vi "UHR-Fleezers Control (host) -Leonardo 04-2018 V2_sym.vi"(0 "Tab Control":T5(tab)=enum."Trap Control (RF)") -> ()   [LabVIEW 2013] (continued)
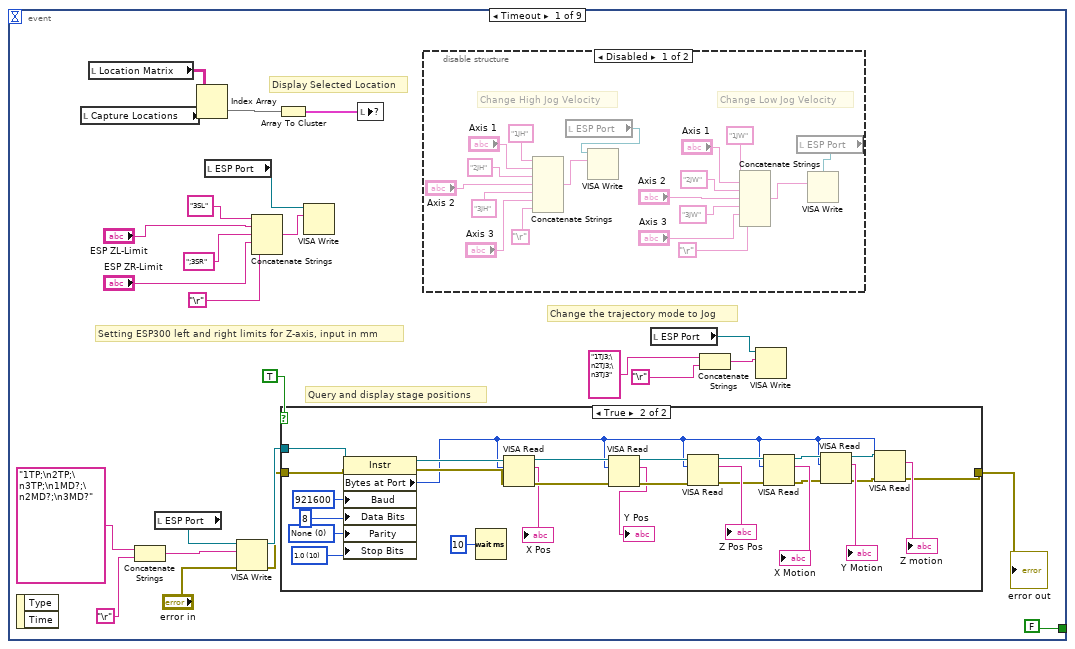
[diagram p2: hidden frame]
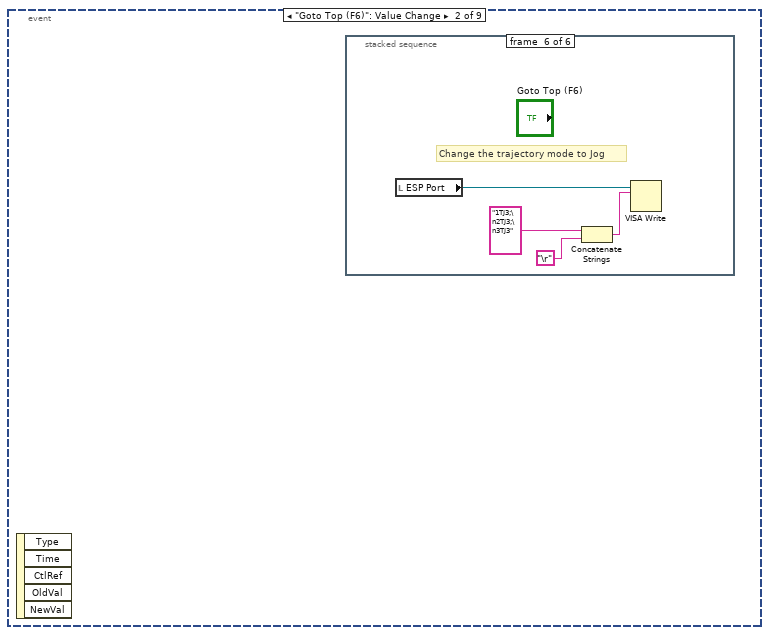
[diagram p5: hidden frame]
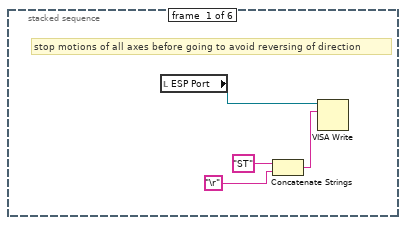
[diagram p6: hidden frame]
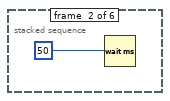
[diagram p7: hidden frame]
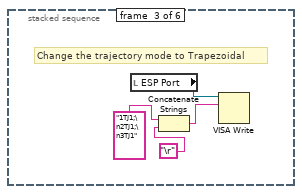
[diagram p8: hidden frame]
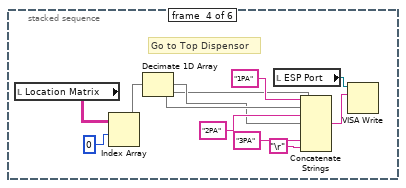
[diagram p9: hidden frame]
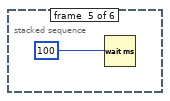
[diagram p10: hidden frame]
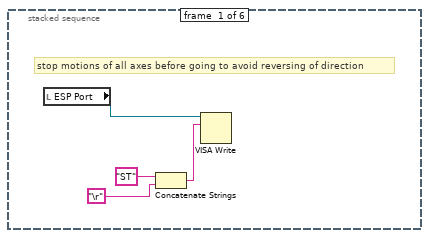
[diagram p11: hidden frame]
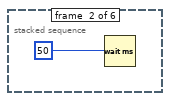
[diagram p12: hidden frame]
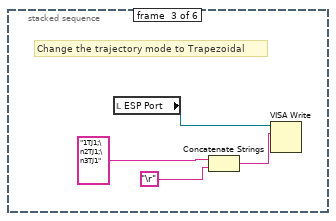
[diagram p13: hidden frame]
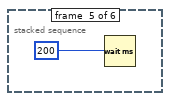
[diagram p14: hidden frame]
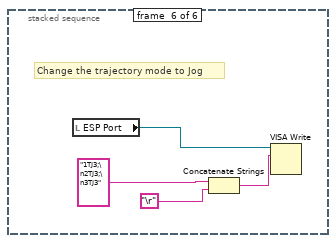
[diagram p15: hidden frame]
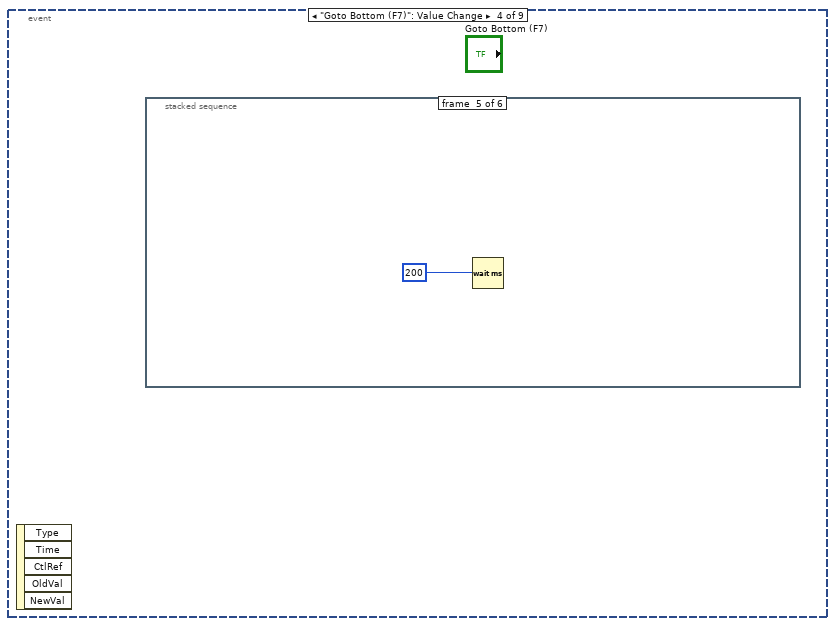
[diagram p16: hidden frame]
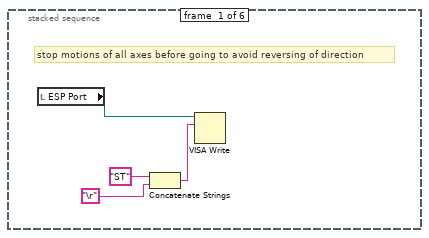
[diagram p17: hidden frame]
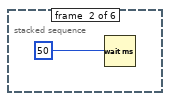
[diagram p18: hidden frame]
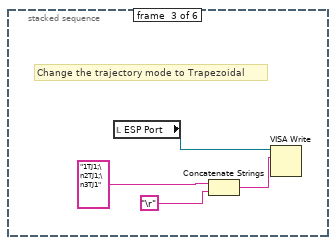
[diagram p19: hidden frame]
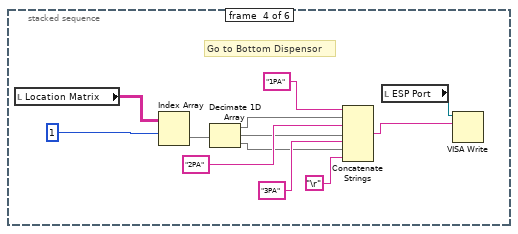
[diagram p20: hidden frame]
                    n2323 = Write to Binary File(file (use dialog)=w3981, data=w3980, 5:FALSE ("prepend array or string size? (T)"), 9:T30."big-endian, network order" ("byte order (0:big-endian, network order)")) -> ()  [unwired: 1 in, 4 out]
                  }
                }
                n2324 = Greater?(x="Save ave N", y=1.0) -> (0:w3950:bool)
                n2325 = Not(x=w3947) -> (.not. x?=w3949:bool)
                n2326 = And(x=w3949, y=w3950) -> (x .and. y?=w3892:bool)
                n2327 = case shown="True" w3892 {
                  tunnel: w3891 -> [w3961 w3972]
                  tunnel: [w3961 w3964] -> w3890
                  tunnel: "Save ave N" -> [_ w3965]
                  frame False {
                  }
                  frame True {
                    w3962 = 2 ("dimension size")
                    n2328 = Array Size(array=w3972) -> (size(s)=w3966:i32)
                    n2329 = Divide(x=w3966, y=w3962) -> (x/y=w3970:dbl)
                    n2330 = Reshape Array(w3972, w3970, w3962) -> (w3971:u64[][])
                    n2331 = Transpose 2D Array(2D array=w3971) -> (transposed array=w3969:u64[][])
                    n2332 = for {
                      tunnel: w3969 -> [w3974] mode=indexing
                      tunnel: [w3973] -> w3963 mode=indexing
                      tunnel: w3965 -> [w3975]
                      workers-P: _ -> [_]
                      n2333 = call "downsample 1D array - U64.vi"("Ave N"=w3975, "Array In"=w3974) -> ("Array Out"=w3973:u64[])  [unwired: 1 in]
                    }
                    n2334 = Transpose 2D Array(2D array=w3963) -> (transposed array=w3968:u64[][])
                    n2335 = Divide(x=w3966, y=w3965) -> (x/y=w3967:dbl)
                    n2336 = Reshape Array(w3968, w3967) -> (w3964:u64[])
                  }
                }
                n2337 = case shown="True" w3892 {
                  tunnel: w3952 -> [w3984 w3996]
                  tunnel: [w3984 w3988] -> w3948
                  tunnel: "Save ave N" -> [_ w3989]
                  tunnel: w3943 -> [_ w3987]
                  frame False {
                    # "don't downsample data for trap calibration"
                  }
                  frame True {
                    n2338 = Array Size(array=w3996) -> (size(s)=w3990:i32)
                    n2339 = Array Size(array=w3987) -> (size(s)=w3986:i32)
                    n2340 = Divide(x=w3990, y=w3986) -> (x/y=w3994:dbl)
                    n2341 = Reshape Array(w3996, w3994, w3986) -> (w3995:i16[][])
                    n2342 = Transpose 2D Array(2D array=w3995) -> (transposed array=w3993:i16[][])
                    n2343 = for {
                      tunnel: w3993 -> [w3999] mode=indexing
                      tunnel: [w3998] -> w3985 mode=indexing
                      tunnel: w3989 -> [w3997]
                      workers-P: _ -> [_]
                      n2344 = call "downsample 1D array - I16.vi"("Ave N"=w3997, "Array In"=w3999) -> ("Array Out"=w3998:i16[])  [unwired: 1 out]
                    }
                    n2345 = Transpose 2D Array(2D array=w3985) -> (transposed array=w3992:i16[][])
                    n2346 = Divide(x=w3990, y=w3989) -> (x/y=w3991:dbl)
                    n2347 = Reshape Array(w3992, w3991) -> (w3988:i16[])
                  }
                }
                n2348 = Index Array(array=w3914, index=1) -> (element=w3917:waveform(dbl))
                n2349 = Index Array(array=w3914, index=0) -> (element=w3919:waveform(dbl))
                n2350 = Unbundle By Name(w3917) -> ("Y"=w3921:dbl[])
                n2351 = Unbundle By Name(w3919) -> ("Y"=w3929:dbl[])
                n2352 = case "Write trap pos. data" shown="True" w3895 {
                  tunnel: w3894 -> [_ w3977]
                  tunnel: w3890 -> [_ w3976]
                  frame False {
                  }
                  frame True {
                    n2353 = Write to Binary File(file (use dialog)=w3977, data=w3976, 5:FALSE ("prepend array or string size? (T)"), 9:T30."big-endian, network order" ("byte order (0:big-endian, network order)")) -> ()  [unwired: 1 in, 4 out]
                  }
                }
                n2354 = Write to Binary File(file (use dialog)=w3955, data=w3948, 5:FALSE ("prepend array or string size? (T)"), 9:T30."big-endian, network order" ("byte order (0:big-endian, network order)")) -> ()  [unwired: 1 in, 4 out]
                n2355 = feedback #26(w3921) -> (w3923:dbl[])
                n2356 = Build Array (concatenate)(w3923, w3921) -> (w3922:dbl[])
                n2357 = Select(t=w3921, s=w3897, f=w3922) -> (s? t:f=w3907:dbl[])
                n2358 = feedback-in #26(w3907) -> ()
                n2359 = feedback #27(w3929) -> (w3942:dbl[])
                n2360 = Build Array (concatenate)(w3942, w3929) -> (w3941:dbl[])
                n2361 = Select(t=w3929, s=w3897, f=w3941) -> (s? t:f=w3916:dbl[])
                n2362 = feedback-in #27(w3916) -> ()
                n2363 = Divide(x=w3956, y=w3957) -> (x/y=w3959:dbl)
                n2364 = Multiply(x=w3959, y=100.0) -> (x*y=w3958:dbl)
                n2365 = Build Array(w3916, w3907) -> (→"Saved APD":dbl[][])
                n2366 = Array Size(array=w3916) -> (size(s)=w3934:i32)
                n2367 = Unbundle By Name(w3936) -> ("Y"=w3940:dbl[])
                n2368 = Subtract(x=w3934, y="N pts to average") -> (x-y=w3910:i32)
                n2369 = Multiply(x="N pts to average", y=u16 2) -> (x*y=w3911:u16)
                n2370 = Subtract(x=w3934, y=w3911) -> (x-y=w3909:i32)
                n2371 = feedback #28(w3940) -> (w3939:dbl[])
                n2372 = Build Array (concatenate)(w3939, w3940) -> (w3938:dbl[])
                n2373 = Select(t=w3940, s=w3897, f=w3938) -> (s? t:f=w3937:dbl[])
                "Trap Delta Graph" <- w3937
                n2374 = feedback-in #28(w3937) -> ()
                n2375 = Array Subset(array=w3916, index=w3910, length="N pts to average") -> (w3933:dbl[])
                n2376 = Array Subset(array=w3916, index=w3909, length="N pts to average") -> (w3932:dbl[])
                n2377 = Array Subset(array=w3907, index=w3910, length="N pts to average") -> (w3913:dbl[])
                n2378 = Array Subset(array=w3907, index=w3909, length="N pts to average") -> (w3912:dbl[])
                n2379 = call-poly <vilib>:"Mean.vi"("X"=w3933) -> ("mean"=w3931:dbl)  [unwired: 1 out]
                n2380 = call-poly <vilib>:"Mean.vi"("X"=w3913) -> ("mean"=w3906:dbl)  [unwired: 1 out]
                n2381 = call-poly <vilib>:"Mean.vi"("X"=w3932) -> ("mean"=w3930:dbl)  [unwired: 1 out]
                n2382 = call-poly <vilib>:"Mean.vi"("X"=w3912) -> ("mean"=w3905:dbl)  [unwired: 1 out]
                n2383 = Subtract(x=w3906, y=w3905) -> (x-y=w3896:dbl)
                "Delta Fl. 2" <- w3896
                n2384 = Subtract(x=w3931, y=w3930) -> (x-y=w3928:dbl)
                "Delta Fl. 1" <- w3928
                n2385 = Initialize Array(w3928, 1 ("dimension size")) -> (w3925:dbl[])
                n2386 = Initialize Array(w3896, 1 ("dimension size")) -> (w3902:dbl[])
                n2387 = feedback #29(w3925) -> (w3926:dbl[])
                n2388 = Build Array (concatenate)(w3926, w3925) -> (w3924:dbl[])
                n2389 = feedback #30(w3902) -> (w3903:dbl[])
                n2390 = Build Array (concatenate)(w3903, w3902) -> (w3901:dbl[])
                n2391 = Select(t=w3925, s=w3897, f=w3924) -> (s? t:f=w3900:dbl[])
                n2392 = feedback-in #29(w3900) -> ()
                n2393 = Select(t=w3902, s=w3897, f=w3901) -> (s? t:f=w3899:dbl[])
                n2394 = feedback-in #30(w3899) -> ()
                n2395 = Build Array(w3900, w3899) -> (→"Save APD Deriv":dbl[][])
              }
            }
            "Progress" <- w3873
            "Progress 2" <- w3873
          }
        }
      }
    }
    n2396 = Divide(x=w2254, y=w2255) -> (x/y=w2245:ext)
    "Trap 2 amplitude" <- w2245
    n2397 = Bundle By Name(cluster=w2508, "Green FB Ch 0"=w2507, "Green FB Ch 1"=w2506) -> (w2492:T49)
    "Green FB Signals (V)" <- w2492
    n2398 = case shown="True" w2247 {
      tunnel: w2246 -> [_ w2597]
      tunnel: w2245 -> [_ w2596]
      frame False {
      }
      frame True {
        w2598 = 50.0
        n2399 = Greater?(x=w2596, y=w2598) -> (0:w2594:bool)
        n2400 = Greater?(x=w2597, y=w2598) -> (0:w2595:bool)
        n2401 = Or(x=w2595, y=w2594) -> (x .or. y?=w2593:bool)
        n2402 = case shown="True" w2593 {
          frame False {
          }
          frame True {
            n2403 = property on="All FB On/Off" class="Bool (strict)"("Val(Sgnl)"=FALSE) -> ()  [unwired: 2 in, 2 out]
            "Feedback overload" <- TRUE
          }
        }
      }
    }
    n2404 = Unbundle By Name(w2492) -> ("Green FB Ch 2"=→"Green FB Plot":dbl)
    n2405 = local read "wait to reset values"() -> (w2576:bool)
    n2406 = Not(x=w2573) -> (.not. x?=w2577:bool)
    n2407 = And(x=w2577, y=w2576) -> (x .and. y?=w2578:bool)
    n2408 = case "Part of MCL raster scanning: returns to initial positions after scan done" shown="True" w2578 {
      tunnel: w2581 -> [w3422 w3429]
      tunnel: [w3422 w3428] -> w2580
      tunnel: w2575 -> [w3421 w3427]
      tunnel: [w3421 w3426] -> w2574
      frame False {
      }
      frame True {
        w3437 = 10.0 ("y")
        w3436 = 32767.0 ("y")
        # "to return scan values\nafter a synchronous \nAOM scan"
        n2409 = local read "AO2"() -> (w3430:dbl)
        n2410 = local read "AO1"() -> (w3431:dbl)
        n2411 = local write "wait to reset values"(FALSE ("wait to reset values")) -> ()
        n2412 = Multiply(x=w3431, y=w3436) -> (x*y=w3433:dbl)
        n2413 = Multiply(x=w3430, y=w3436) -> (x*y=w3435:dbl)
        n2414 = Divide(x=w3433, y=w3437) -> (x/y=w3432:dbl)
        n2415 = Divide(x=w3435, y=w3437) -> (x/y=w3434:dbl)
        n2416 = To Word Integer(number=w3432) -> (16bit integer=w3438:i16)
        n2417 = To Word Integer(number=w3434) -> (16bit integer=w3439:i16)
        n2418 = local read "Total Counts (ticks)"() -> (w3423:u32)
        n2419 = xnode "Read/Write Control"("FPGA VI Reference In"=w3429, "error in"=w3427, "AO1 (Y)"=w3438, "AO2 (X)"=w3439, "MCL count"=w3423) -> ("FPGA VI Reference Out"=w3428:T20, "error out"=w3426:errorcluster)
        n2420 = local read "Scan Range (V)\n(of steps)"() -> (w3424:dbl)
        n2421 = property on="Scan Range (V)\n(of steps)" class="DigNum (strict)"("Val(Sgnl)"=w3424) -> ()  [unwired: 2 in, 2 out]
      }
    }
    n2422 = node-c288() -> ()  [unwired: 2 out]
  }
  n2423 = node-c288(3 ("Processor")) -> (w108:T25)  [unwired: 3 out]
  n2424 = timed-loop "Oscillate AOD (debugging)" {
    tunnel: w61 -> [w4001]
    tunnel: [w4000] -> w72
    timing: w108 -> [_]
    timing-out: [_] -> w107
    stop <- w4000 stop-if-true
    n2425 = node-c288() -> ()  [unwired: 2 out]
    n2426 = event shown="[0] \"Oscillate Set 2\", \"Fish for Tether\": Value Change" {
      selector: _ -> [_ _ _]
      dyn-events: _ -> [_ _ _]
      timeout: _ -> [_ _ _]
      tunnel: w4001 -> [w4008 _ _]
      tunnel: [FALSE ("Stop All") _ w4276] -> w4000
      event "Oscillate Set 2", "Fish for Tether": Value Change {
        n2427 = event-data() -> ()  [unwired: 6 out]
        n2428 = local read "Oscillate Set 2"() -> (w4007:bool)
        n2429 = Or(x=w4007, y="Fish for Tether") -> (x .or. y?=w4005:bool)
        n2430 = case shown="True" w4005 {
          tunnel: w4008 -> [_ w4011]
          tunnel: "Fish for Tether" -> [_ w4010]
          frame False {
          }
          frame True {
            n2431 = case shown="True" w4010 {
              frame False {
              }
              frame True {
                n2432 = local write "Scan axis 2"(TRUE) -> ()
                n2433 = local write "Tether"(FALSE ("Tether")) -> ()
              }
            }
            n2434 = node-c288("Period") -> (w4013:T25)  [unwired: 3 out]
            n2435 = timed-loop "Oscillate AOD" {
              timing: w4013 -> [_]
              timing-out: [_] -> w4012
              tunnel: w4011 -> [w4023]
              tunnel: w4010 -> [w4022]
              i -> [w4025]
              stop <- w4021 stop-if-true
              n2436 = node-c288() -> (w4024:i64)  [unwired: 1 out]
              n2437 = flat-sequence {
                tunnel: w4025 -> [w4051]
                tunnel: w4024 -> [w4050]
                tunnel: w4023 -> [w4034]
                tunnel: w4022 -> [w4036]
                tunnel: [w4036] -> w4020
                tunnel: [w4035] -> w4019
                tunnel: [w4033] -> w4018
                tunnel: [w4030] -> w4016
                tunnel: w4020 -> [w4087]
                tunnel: w4019 -> [w4085]
                tunnel: w4018 -> [w4084]
                tunnel: [w4083] -> w4017
                tunnel: w4016 -> [w4082]
                tunnel: [w4151] -> w4021
                tunnel: w4017 -> [w4149]
                frame #0 {
                  n2438 = Divide(x=w4050, y=i64 1000) -> (x/y=w4045:dbl)
                  n2439 = Multiply(x=w4045, y=w4051) -> (x*y=w4047:dbl)
                  n2440 = Multiply(x="Osc. freq. (Hz)", y=6.283185307179586) -> (x*y=w4048:dbl)
                  n2441 = Multiply(x=w4048, y=w4047) -> (x*y=w4032:dbl)
                  n2442 = local read "BD 1 Frequency 2 (MHz)"() -> (w4029:dbl)
                  n2443 = local read "BD 1 Frequency 1 (MHz)"() -> (w4026:dbl)
                  n2444 = case shown="True" w4036 {
                    tunnel: w4032 -> [w4057 w4064]
                    tunnel: w4029 -> [_ w4074]
                    tunnel: [w4054 w4058] -> w4037
                    tunnel: [FALSE w4067] -> w4033
                    tunnel: [0.0 w4060] -> w4030
                    tunnel: w4026 -> [_ w4059]
                    frame False {
                      n2445 = Sine(x=w4057) -> (sin(x)=w4055:dbl)
                      n2446 = Multiply(x=w4055, y="Osc. amp. (MHz)") -> (x*y=w4054:dbl)
                    }
                    frame True {
                      n2447 = Cosine(x=w4064) -> (cos(x)=w4077:dbl)
                      n2448 = Subtract(x=w4074, y=w4059) -> (x-y=w4073:dbl)
                      n2449 = Decrement(x=w4077) -> (x-1=w4076:dbl)
                      n2450 = Subtract(x=w4073, y="Closest Delta (MHz)") -> (x-y=w4070:dbl)
                      n2451 = Divide(x=w4076, y=2.0) -> (x/y=w4071:dbl)
                      n2452 = Multiply(x=w4071, y=w4070) -> (x*y=w4058:dbl)
                      n2453 = local read "Vec Mean of T1 T2"() -> (w4066:dbl[])
                      n2454 = Greater?(x=w4066, y="Stop F (pN)") -> (0:w4068:bool[])
                      n2455 = Or Array Elements(Boolean array=w4068) -> (logical OR=w4067:bool)
                      n2456 = Divide(x=w4064, y=6.283185307179586) -> (x/y=w4063:dbl)
                      n2457 = Round Toward +Infinity(x=w4063) -> (ceil(x): smallest int >= x=w4060:dbl)
                      "Attempts" <- w4060
                      n2458 = Greater?(x=w4060, y="Attempt Limit") -> (0:w4062:bool)
                      n2459 = case shown="True" w4062 {
                        frame False {
                        }
                        frame True {
                          n2460 = local write "Fish for Tether"(FALSE ("Fish for Tether")) -> ()
                          n2461 = call <vilib>:"Beep.vi"() -> ()  [unwired: 3 in, 9 out]
                          n2462 = local read "Messages"() -> (w4079:string)
                          n2463 = call "Update messages.vi"("Message to add"="Tether fishing timeout." ("Messages"), "Old message string"=w4079) -> ("New message string"=→"Messages":string)
                        }
                      }
                    }
                  }
                  n2464 = local read "Y RF Frequency Limits (MHz)"() -> (w4038:T16)
                  n2465 = local read "X RF Frequency Limits (MHz)"() -> (w4039:T16)
                  n2466 = local read "BD 1 Frequency 3 (MHz)"() -> (w4044:dbl)
                  n2467 = local read "BD 2 Frequency 2 (MHz)"() -> (w4028:dbl)
                  n2468 = Select(t=w4029, s="Scan axis 2", f=w4028) -> (s? t:f=w4040:dbl)
                  n2469 = Add(x=w4037, y=w4040) -> (x+y=w4035:dbl)
                  n2470 = Select(t=w4035, s="Scan axis 2", f=w4029) -> (s? t:f=w4027:dbl)
                  n2471 = Select(t=w4028, s="Scan axis 2", f=w4035) -> (s? t:f=w4042:dbl)
                  n2472 = local read "BD 2 Frequency 3 (MHz)"() -> (w4043:dbl)
                  n2473 = call "set RF board frequency - interlace.vi"("Board 2 Frequency Limits"=w4038, "Board 1 Frequency Limits"=w4039, "FPGA VI Reference In"=w4034, "Board 2 Frequency 3 (MHz)"=w4043, "Board 1 Frequency 3 (MHz)"=w4044, "Board 2 Frequency 2 (MHz)"=w4028, "Board 2 Frequency 1 (MHz)"=w4042, "Board 1 Frequency 2 (MHz)"=w4027, "Board 1 Frequency 1  (MHz)"=w4026) -> ()  [unwired: 1 in, 2 out]
                }
                frame #1 {
                  n2474 = And(x=w4087, y=w4084) -> (x .and. y?=w4086:bool)
                  n2475 = case "Only if were fishing and now formed tether" shown="True" w4086 {
                    tunnel: w4085 -> [w4089 w4101]
                    tunnel: [w4088 w4100] -> w4083
                    tunnel: w4082 -> [_ w4096]
                    frame False {
                      n2476 = local read "Fish for Tether"() -> (w4088:bool)
                      n2477 = case shown="True" w4088 {
                        tunnel: w4089 -> [_ _]
                        frame False {
                        }
                        frame True {
                        }
                      }
                    }
                    frame True {
                      w4100 = FALSE ("Fish for Tether")
                      n2478 = call <vilib>:"Beep.vi"() -> ()  [unwired: 3 in, 9 out]
                      n2479 = Number To Decimal String(number=w4096, width (-)=i16 1) -> (decimal integer string=w4094:string)
                      n2480 = case shown="\"2\", \"3\", \"4\", \"5\", \"6\"" "Then..." {
                        selector: "Then..." -> [_ w4104]
                        tunnel: w4101 -> [w4103 _]
                        frame "1", Default {
                          # "do nothing"
                          n2481 = property on="BD 1 Frequency 1 (MHz)" class="DigNum (strict)"("Val(Sgnl)"=w4103) -> ()  [unwired: 2 in, 2 out]
                        }
                        frame "2", "3", "4", "5", "6" {
                          n2482 = flat-sequence {
                            tunnel: w4104 -> [w4106]
                            frame #0 {
                              n2483 = property on="Trap Delta (MHz)" class="DigNum (strict)"("Val(Sgnl)"="Move to Delta 1 (MHz)") -> ()  [unwired: 2 in, 2 out]
                            }
                            frame #1 {
                              n2484 = case shown="\"5\", \"6\"" w4106 {
                                selector: w4106 -> [w4109 w4119 _]
                                frame "3", "4" {
                                n2485 = flat-sequence {
                                tunnel: w4109 -> [w4110]
                                tunnel: [w4110] -> w4107
                                tunnel: [w4112] -> w4108
                                tunnel: w4107 -> [w4112]
                                tunnel: w4108 -> [w4116]
                                frame #0 {
                                n2486 = property on="Green Laser ON/Interlacing" class="Bool (strict)"("Val(Sgnl)"=TRUE ("Value (Signaling)")) -> ()  [unwired: 2 in, 2 out]
                                }
                                frame #1 {
                                n2487 = Multiply(x="Wait Before Save (s)", y=u32 1000 ("x")) -> (x*y=w4114:u32)
                                n2488 = Wait (ms)(milliseconds to wait=w4114) -> ()  [unwired: 1 out]
                                }
                                frame #2 {
                                n2489 = property on="Start Saving" class="Bool (strict)"("Value"=TRUE ("Start Saving")) -> ()  [unwired: 2 in, 2 out]
                                n2490 = case shown="Default" w4116 {
                                frame Default {
                                }
                                frame "4" {
                                n2491 = property on="Fl. Triggered..." class="Bool (strict)"("Val(Sgnl)"=TRUE ("Value (Signaling)")) -> ()  [unwired: 2 in, 2 out]
                                }
                                }
                                }
                                }
                                }
                                frame "5", "6" {
                                n2492 = stacked-sequence {
                                tunnel: w4119 -> [_ _ _ _ _ _ _ _ w4136 _ _]
                                frame #0 {
                                n2493 = Replace Array Subset(array=u32[] [0] ("Index Values"), new element="Raster Set Upon Tether", index=0) -> (w4120:u32[])
                                n2494 = property on="Saved AOD Raster Scan Parameter Sets" class="Arr (strict)"("Index Values"=w4120) -> ()  [unwired: 2 in, 2 out]
                                }
                                frame #1 {
                                n2495 = Wait (ms)(milliseconds to wait=u32 500) -> ()  [unwired: 1 out]
                                }
                                frame #2 {
                                n2496 = property on="Load parameters" class="Bool (strict)"("Val(Sgnl)"=TRUE ("Value (Signaling)")) -> ()  [unwired: 2 in, 2 out]
                                }
                                frame #3 {
                                n2497 = Wait (ms)(milliseconds to wait=u32 500) -> ()  [unwired: 1 out]
                                }
                                frame #4 {
                                n2498 = property on="Trap Raster Scan" class="Bool (strict)"("Val(Sgnl)"=TRUE ("Value (Signaling)")) -> ()  [unwired: 2 in, 2 out]
                                }
                                frame #5 {
                                n2499 = Wait (ms)(milliseconds to wait=u32 2000) -> ()  [unwired: 1 out]
                                }
                                frame #6 {
                                n2500 = while {
                                stop <- w4131 stop-if-true
                                n2501 = local read "Raster Scanning..."() -> (w4130:bool)
                                n2502 = local read "Saving..."() -> (w4133:bool)
                                n2503 = Wait (ms)(milliseconds to wait=u32 100) -> ()  [unwired: 1 out]
                                n2504 = Not(x=w4133) -> (.not. x?=w4132:bool)
                                n2505 = Not(x=w4130) -> (.not. x?=w4129:bool)
                                n2506 = And(x=w4132, y=w4129) -> (x .and. y?=w4131:bool)
                                }
                                }
                                frame #7 {
                                n2507 = property on="Trap Delta (MHz)" class="DigNum (strict)"("Val(Sgnl)"="Move to Delta 2 (MHz)") -> ()  [unwired: 2 in, 2 out]
                                }
                                frame #8 {
                                n2508 = local read "Tether"() -> (w4137:bool)
                                n2509 = case shown="True" w4137 {
                                tunnel: w4136 -> [_ w4138]
                                frame False {
                                }
                                frame True {
                                n2510 = flat-sequence {
                                tunnel: w4138 -> [w4140]
                                frame #0 {
                                n2511 = Wait (ms)(milliseconds to wait=u32 500) -> ()  [unwired: 1 out]
                                }
                                frame #1 {
                                n2512 = case shown="\"6\"" w4140 {
                                frame Default {
                                }
                                frame "6" {
                                n2513 = property on="Green Laser ON/Interlacing" class="Bool (strict)"("Val(Sgnl)"=TRUE ("Green Laser ON/Interlacing")) -> ()  [unwired: 2 in, 2 out]
                                }
                                }
                                }
                                frame #2 {
                                n2514 = Wait (ms)(milliseconds to wait=u32 500) -> ()  [unwired: 1 out]
                                }
                                frame #3 {
                                n2515 = local write "Start Saving"("Save at end (5, 6)") -> ()
                                }
                                }
                                }
                                }
                                }
                                frame #9 {
                                n2516 = local read "Bead Sep. Int. Time (s)"() -> (w4146:dbl)
                                n2517 = Multiply(x=w4146, y=1000.0) -> (x*y=w4145:dbl)
                                n2518 = Wait (ms)(milliseconds to wait=w4145) -> ()  [unwired: 1 out]
                                }
                                frame #10 {
                                n2519 = property on="Rescale on Mean" class="Bool (strict)"("Val(Sgnl)"=TRUE ("Value (Signaling)")) -> ()  [unwired: 2 in, 2 out]
                                }
                                }
                                }
                                frame "2", Default {
                                }
                              }
                            }
                          }
                        }
                      }
                      n2520 = Concatenate Strings("Formed tether in ", w4094, " attempt(s)." ("string")) -> (w4091:string)
                      n2521 = local read "Messages"() -> (w4098:string)
                      n2522 = local write "Fish for Tether"(w4100) -> ()
                      n2523 = call "Update messages.vi"("Message to add"=w4091, "Old message string"=w4098) -> ("New message string"=w4097:string)
                      n2524 = local write "Messages"(w4097) -> ()
                      n2525 = Get Date/Time In Seconds() -> (seconds since 1Jan1904=→"Time tether formed":timestamp)
                      "Tether" <- "Tether Alarm?"
                    }
                  }
                }
                frame #2 {
                  n2526 = local read "Oscillate Set 2"() -> (w4150:bool)
                  n2527 = local read "Stop All"() -> (w4152:bool)
                  n2528 = Not Or(1:w4149, 2:w4150) -> (0:w4148:bool)
                  n2529 = Compound Arithmetic op=OR(w4152, w4148) -> (w4151:bool)
                }
              }
              n2530 = node-c288() -> ()  [unwired: 2 out]
            }
            n2531 = node-c288(w4012) -> ()  [unwired: 1 out]
          }
        }
      }
      event "Fl. Triggered...": Value Change {
        n2532 = event-data() -> ()  [unwired: 7 out]
        n2533 = case shown="True" "Fl. Triggered..." {
          frame False {
          }
          frame True {
            n2534 = node-c288() -> (w4164:T25)  [unwired: 4 out]
            n2535 = timed-loop {
              timing: w4164 -> [_]
              timing-out: [_] -> w4163
              tunnel: "Action" -> [w4168]
              shift-right: [w4165] -> _
              shift-left: u8 255 -> [w4167]
              stop <- w4169 stop-if-true
              n2536 = node-c288() -> ()  [unwired: 2 out]
              n2537 = flat-sequence {
                tunnel: w4168 -> [w4181]
                tunnel: w4167 -> [w4178]
                tunnel: [w4177] -> w4166
                tunnel: [w4267] -> w4169
                tunnel: w4166 -> [w4266]
                tunnel: [w4266] -> w4165
                frame #0 {
                  n2538 = local read "Delta Fl. 2"() -> (w4172:dbl)
                  n2539 = local read "Delta Fl. 1"() -> (w4173:dbl)
                  n2540 = Select(t=w4173, s="APD to Watch", f=w4172) -> (s? t:f=w4171:dbl)
                  n2541 = Multiply(x="Fl. Delta Thresh. (kHz)", y=1000.0) -> (x*y=w4180:dbl)
                  n2542 = Greater?(x=w4171, y=w4180) -> (0:w4175:bool)
                  n2543 = Or(x="Force Yank", y=w4175) -> (x .or. y?=w4176:bool)
                  n2544 = case shown="True" w4176 {
                    tunnel: w4181 -> [_ w4191]
                    tunnel: w4178 -> [w4183 w4187]
                    tunnel: [w4183 w4184] -> w4177
                    frame False {
                    }
                    frame True {
                      n2545 = flat-sequence {
                        tunnel: w4188 -> [w4197]
                        tunnel: [w4197] -> w4192
                        tunnel: w4191 -> [w4196]
                        tunnel: [w4196] -> w4190
                        tunnel: [w4195] -> w4189
                        tunnel: w4187 -> [w4194]
                        tunnel: [w4193] -> w4186
                        tunnel: w4192 -> [w4222]
                        tunnel: w4190 -> [w4221]
                        tunnel: w4189 -> [w4220]
                        tunnel: w4186 -> [w4219]
                        tunnel: [w4219] -> w4185
                        tunnel: w4185 -> [w4264]
                        tunnel: [w4264] -> w4184
                        frame #0 {
                          n2546 = call <vilib>:"Beep.vi"() -> ()  [unwired: 3 in, 9 out]
                          n2547 = local write "Waiting"(FALSE ("Waiting")) -> ()
                          n2548 = Increment(x=w4194) -> (x+1=w4193:u8)
                          n2549 = case shown="\"Yank\"" w4196 {
                            tunnel: w4193 -> [_ _ w4203]
                            frame "Image" {
                              n2550 = property on="Confocal Image" class="Bool (strict)"("Val(Sgnl)"=TRUE ("Value (Signaling)")) -> ()  [unwired: 2 in, 2 out]
                            }
                            frame "Alarm", Default {
                            }
                            frame "Yank" {
                              n2551 = flat-sequence {
                                tunnel: w4203 -> [w4206]
                                tunnel: [w4205] -> w4202
                                tunnel: ["N Array El"] -> w4201
                                tunnel: w4202 -> [w4216]
                                tunnel: w4201 -> [w4212]
                                frame #0 {
                                n2552 = Multiply(x="Yank Delay (s)", y=1000.0) -> (x*y=w4209:dbl)
                                n2553 = Quotient & Remainder(x=w4206, y="N Array El") -> (x-y*floor(x/y)=w4205:u8)  [unwired: 1 out]
                                n2554 = Wait (ms)(milliseconds to wait=w4209) -> ()  [unwired: 1 out]
                                }
                                frame #1 {
                                n2555 = Random Number (0-1)() -> (number: 0 to 1=w4213:dbl)
                                n2556 = Multiply(x=w4212, y=w4213) -> (x*y=w4211:dbl)
                                n2557 = Round Toward -Infinity(1:w4211) -> (0:w4210:dbl)
                                n2558 = Select(t=w4210, s="Random Choice", f=w4216) -> (s? t:f=w4214:dbl)
                                n2559 = Index Array(array="Yank to Delta Array (MHz)", index=w4214) -> (element=w4217:dbl)
                                n2560 = property on="Trap Delta (MHz)" class="DigNum (strict)"("Val(Sgnl)"=w4217) -> ()  [unwired: 2 in, 2 out]
                                }
                              }
                            }
                          }
                          n2561 = local read "Time (s)"() -> (w4195:dbl)
                          "Fl. High" <- TRUE ("Yanking")
                        }
                        frame #1 {
                          n2562 = node-c288() -> (w4224:T25)  [unwired: 4 out]
                          n2563 = timed-loop {
                            timing: w4224 -> [_]
                            timing-out: [_] -> w4223
                            tunnel: w4222 -> [w4240]
                            tunnel: w4221 -> [w4238]
                            tunnel: w4220 -> [w4237]
                            stop <- w4239 stop-if-true
                            n2564 = node-c288() -> ()  [unwired: 2 out]
                            n2565 = local read "Fl. Delta Thresh. (kHz)"() -> (w4232:dbl)
                            n2566 = local read "Fl. Triggered..."() -> (w4241:bool)
                            n2567 = local read "Delta Fl. 1"() -> (w4228:dbl)
                            n2568 = local read "Delta Fl. 2"() -> (w4226:dbl)
                            n2569 = local read "Stop All"() -> (w4235:bool)
                            n2570 = local read "APD to Watch"() -> (w4227:bool)
                            n2571 = Select(t=w4228, s=w4227, f=w4226) -> (s? t:f=w4225:dbl)
                            n2572 = Not(x=w4241) -> (.not. x?=w4236:bool)
                            n2573 = Multiply(x=w4232, y=1000.0) -> (x*y=w4231:dbl)
                            n2574 = Negate(x=w4231) -> (-x=w4230:dbl)
                            n2575 = Less?(x=w4225, y=w4230) -> (x < y?=w4234:bool)
                            n2576 = Compound Arithmetic op=OR(w4234, w4235, w4236, "Force Reset") -> (w4239:bool)
                            n2577 = case shown="True" w4239 {
                              tunnel: w4240 -> [_ w4252]
                              tunnel: w4238 -> [_ w4251]
                              tunnel: w4237 -> [_ w4249]
                              frame False {
                              }
                              frame True {
                                n2578 = case shown="\"Yank\"" w4251 {
                                tunnel: w4252 -> [_ w4253]
                                frame "Image", Default {
                                }
                                frame "Yank" {
                                n2579 = flat-sequence {
                                tunnel: [w4258] -> w4254
                                tunnel: w4253 -> [w4258]
                                tunnel: w4254 -> [w4259]
                                frame #0 {
                                n2580 = local read "Yank Delay (s)"() -> (w4257:dbl)
                                n2581 = Multiply(x=w4257, y=1000.0) -> (x*y=w4255:dbl)
                                n2582 = Wait (ms)(milliseconds to wait=w4255) -> ()  [unwired: 1 out]
                                }
                                frame #1 {
                                n2583 = property on="Trap Delta (MHz)" class="DigNum (strict)"("Val(Sgnl)"=w4259) -> ()  [unwired: 2 in, 2 out]
                                }
                                }
                                }
                                }
                                n2584 = local read "Time (s)"() -> (w4250:dbl)
                                n2585 = Subtract(x=w4250, y=w4249) -> (x-y=w4246:dbl)
                                "Duration (s)" <- w4246
                                n2586 = Number To Decimal String(number=w4246, width (-)=i16 0) -> (decimal integer string=w4244:string)
                                n2587 = Concatenate Strings(w4244, " s fluorescence event." ("string")) -> (w4242:string)
                                n2588 = local read "Messages"() -> (w4248:string)
                                n2589 = call "Update messages.vi"("Message to add"=w4242, "Old message string"=w4248) -> ("New message string"=w4247:string)
                                n2590 = call <vilib>:"Beep.vi"() -> ()  [unwired: 3 in, 9 out]
                                n2591 = local write "Messages"(w4247) -> ()
                              }
                            }
                            n2592 = node-c288() -> ()  [unwired: 2 out]
                          }
                          n2593 = node-c288(w4223) -> ()  [unwired: 1 out]
                        }
                        frame #2 {
                          n2594 = local write "Fl. High"(FALSE ("Yanking")) -> ()
                        }
                      }
                      n2595 = local read "Trap Delta (MHz)"() -> (w4188:dbl)
                    }
                  }
                }
                frame #1 {
                  n2596 = local read "Stop All"() -> (w4270:bool)
                  n2597 = local read "Fl. Triggered..."() -> (w4268:bool)
                  n2598 = Not(x=w4268) -> (.not. x?=w4269:bool)
                  n2599 = Or(x=w4269, y=w4270) -> (x .or. y?=w4267:bool)
                  n2600 = Not(x=w4267) -> (.not. x?=→"Waiting":bool)
                }
              }
              n2601 = node-c288() -> ()  [unwired: 2 out]
            }
            n2602 = node-c288(w4163) -> ()  [unwired: 1 out]
          }
        }
      }
      event "Stop All": Value Change {
        n2603 = event-data() -> ()  [unwired: 7 out]
        n2604 = local read "Stop All"() -> (w4276:bool)
      }
    }
    n2605 = node-c288() -> ()  [unwired: 2 out]
  }
  n2606 = node-c288(w107) -> ()  [unwired: 1 out]
  n2607 = node-c288(w194) -> ()  [unwired: 1 out]
  n2608 = flat-sequence "@Alex - Set stage to 0,0,0 on exit" {
    tunnel: w2 -> [w4278]
    tunnel: [w4277] -> w1
    frame #0 {
      n2609 = local read "ESP Port"() -> (w4282:refnum<visa-resource-name>)
      n2610 = Concatenate Strings("1PA0;\n2PA0;\n3PA0" ("write buffer"), "\r") -> (w4279:string)
      n2611 = VISA Write(VISA resource name=w4282, write buffer=w4279, error in (no error)=w4278) -> (error out=w4277:errorcluster)  [unwired: 2 out]
    }
  }
  n2612 = flat-sequence {
    tunnel: w69 -> [w4287]
    tunnel: [w4286] -> w75
    tunnel: [w4283] -> w74
    tunnel: w73 -> [_]
    tunnel: w72 -> [_]
    tunnel: w71 -> [_]
    tunnel: w70 -> [_]
    tunnel: w1 -> [w4284]
    tunnel: w75 -> [w4290]
    tunnel: w74 -> [w4289]
    frame #0 {
      w4285 = FALSE ("APD to FIFO")
      n2613 = xnode "Read/Write Control"("FPGA VI Reference In"=w4287, "error in"=w4284, "APD to FIFO"=w4285, "AI to FIFO"=w4285) -> ("FPGA VI Reference Out"=w4286:T20, "error out"=w4283:errorcluster)
    }
    frame #1 {
      n2614 = xnode "Invoke Method"("FPGA VI Reference In"=w4290, "error in"=w4289) -> ("FPGA VI Reference Out"=w4288:T20)  [unwired: 1 out]
      n2615 = xnode "Close FPGA VI Reference"("FPGA VI Reference In"=w4288) -> ()  [unwired: 1 in, 1 out]
    }
  }
